vi "Reconnect VISA.vi"(8 "error in":errorcluster, 11 "VISA resource name":refnum<visa-resource-name>) -> (0 "error out":errorcluster, 3 "VISA resource name 2":refnum<visa-resource-name>)   [LabVIEW 2024]
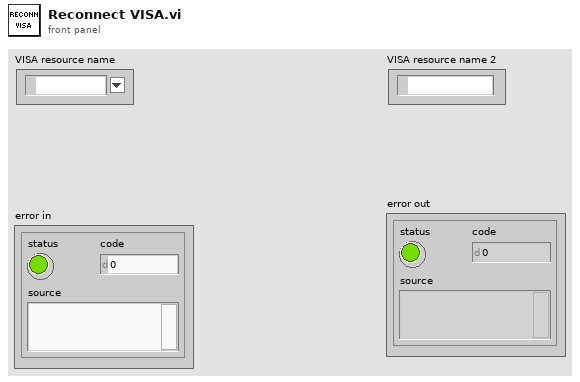
[diagram p1: front panel]
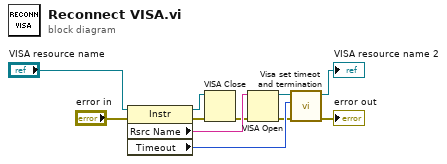
[diagram p0: block diagram]
diagram:
  n1 = property class="Instr"(reference="VISA resource name", error in="error in") -> (reference out=w2:refnum<visa-resource-name>, error out=w3:errorcluster, "Rsrc Name"=w9:string, "Timeout"=w8:u32)
  n2 = VISA Close(VISA resource name=w2, error in (no error)=w3) -> (error out=w1:errorcluster)
  n3 = VISA Open(error in (no error)=w1, VISA resource name=w9) -> (VISA resource name=w7:refnum<visa-resource-name>, error out=w6:errorcluster)  [unwired: 3 in]
  n4 = call "Visa set timeot and termination.vi"("error in (no error)"=w6, "Timeout Value"=w8, "VISA resource name"=w7) -> ("error out"=→"error out":errorcluster, "VISA resource name out"=→"VISA resource name 2":refnum<visa-resource-name>)  [unwired: 4 in, 3 out]
